vi "Fibonacci.vi"(11 "Num":i32=100) -> (3 "Fibonacci":i32[](array[numeric]))   [LabVIEW 2013]
doc: "a0=1\na1=1\na(n+2)=a(n)+a(n+1)\n1、1、2、3、5、8、13......"
panel:
  # "Fibonacci"
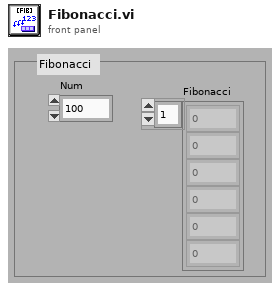
[diagram p1: front panel]
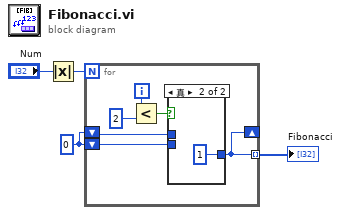
[diagram p0: block diagram]
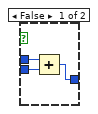
[diagram p2: hidden frame]
diagram:
  w2 = 0
  n1 = Absolute Value(x="Num") -> (abs(x)=w3:i32)
  n2 = for {
    N: w3 -> [_]
    shift-right: [w5] -> _
    shift-left: w2 -> [w7]
    shift-left: w2 -> [w6]
    tunnel: [w5] -> w1 mode=indexing
    i -> [w10]
    n3 = Less?(x=w10, y=2) -> (x < y?=w8:bool)
    n4 = case shown="真" w8 {
      tunnel: w7 -> [w13 _]
      tunnel: w6 -> [w12 _]
      tunnel: [w11 1] -> w5
      frame False {
        n5 = Add(x=w13, y=w12) -> (x+y=w11:i32)
      }
      frame True {
      }
    }
  }
  "Fibonacci" <- w1
